vi "Statistics Find Frequency and Index.vi"(9 "Frequency Channel Name":string="Frequency", 10 "MHz":dbl, 11 "Channel Data":T1[](array[typedef])) -> (0 "In Range?":bool, 1 "Frequency":dbl, 2 "Frequency Index":dbl, 3 "Frequency Array":dbl[](array[numeric]))   [LabVIEW 2011]
uses:
  TDMS/TDMS Channel (Sxx).ctl
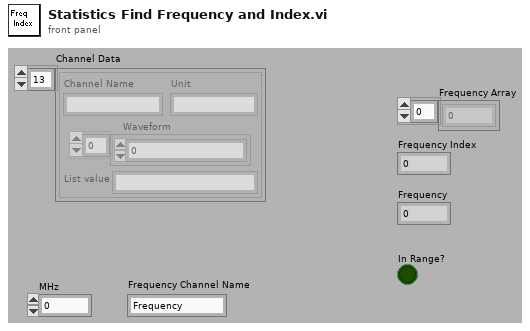
[diagram p1: front panel]
types:
  T1 = typedef "TDMS Channel (Sxx).ctl" = cluster{"Channel Name":string, "Waveform":dbl[], "Unit":string, "List value":string}
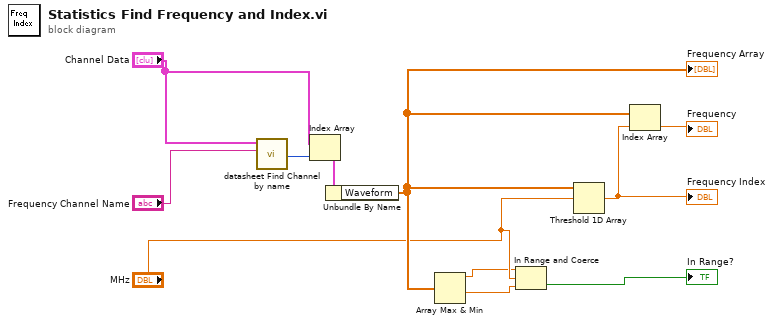
[diagram p0: block diagram]
diagram:
  n1 = call "datasheet Find Channel by name.vi"("Channel Name"="Frequency Channel Name", "Channel Data"="Channel Data") -> ("index of element"=w10:i32)  [unwired: 9 out]
  n2 = Index Array(array="Channel Data", index=w10) -> (element=w9:T1)
  n3 = Unbundle By Name(w9) -> ("Waveform"=w5:dbl[])
  "Frequency Array" <- w5
  n4 = Array Max & Min(array=w5) -> (max value=w3:dbl, min value=w2:dbl)  [unwired: 2 out]
  n5 = In Range and Coerce(upper limit=w3, x="MHz", lower limit=w2) -> (In Range?=→"In Range?":bool)  [unwired: 1 out]
  n6 = Threshold 1D Array(2:"MHz", 3:w5) -> (0:w8:dbl)  [unwired: 1 out]
  "Frequency Index" <- w8
  n7 = Index Array(array=w5, index=w8) -> (element=→"Frequency":dbl)
